vi "Initialize Offsets.vi"() -> (0 "Transactions":T1[](array[typedef]))   [LabVIEW 2013]
uses:
  Data Access Objects/Application/Number Of LBCBs.ctl
  Global Data/Transactions/Dataset Source.ctl
  Global Data/Transactions/Dataset Type.ctl
  Apps/Yes No Button.ctl
  Global Data/Transactions/Dataset Transaction Id.ctl
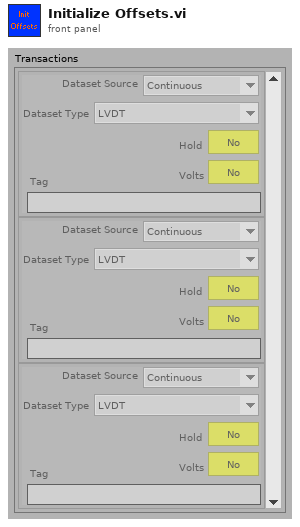
[diagram p1: front panel]
types:
  T1 = typedef "Dataset Transaction Id.ctl" = cluster{"Dataset Source":T2, "Dataset Type":T3, "Hold":T4, "Volts":T4, "Tag":string}
  T2 = typedef "Dataset Source.ctl" = enum16{"Continuous", "Hold", "ED", "Volts", "Offsets", "Increments"}
  T3 = typedef "Dataset Type.ctl" = enum16{"LVDT", "Load Cell", "Actuator Command", "Servo Error", "Displacement Command", "Displacement", "Force"}
  T4 = typedef "Yes No Button.ctl" = bool
  T5 = typedef "Number Of LBCBs.ctl" = enum16{"1", "2"}
  T6 = typedef "Dataset Source.ctl" = enum16{"Continuous", "Hold", "ED", "Volts", "Offsets"}
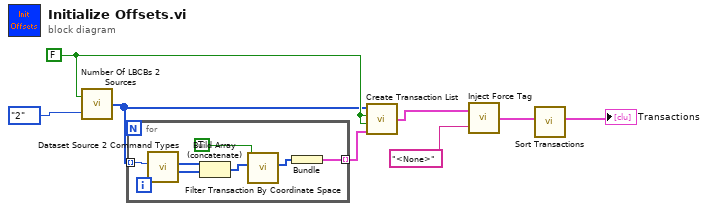
[diagram p0: block diagram]
diagram:
  w7 = FALSE ("Combined LBCBs")
  n1 = call "Number Of LBCBs 2 Sources.vi"("Number of LBCBs"=Number_Of_LBCBs."2", "Combined LBCBs"=w7) -> ("Sources"=w3:T6[])
  n2 = for {
    tunnel: w3 -> [w15] mode=indexing
    tunnel: [w9] -> w2 mode=indexing
    n3 = call "Dataset Source 2 Command Types.vi"("Dataset Source"=w15) -> ("No Command Types Out"=w13:T3[], "Command Types"=w14:T3[])  [unwired: 9 in]
    n4 = Build Array (concatenate)(w14, w13) -> (w12:T3[])
    n5 = call "Filter Transaction By Coordinate Space.vi"("Types In"=w12, "Coordinate Space"=TRUE) -> ("Types Out"=w10:T3[])  [unwired: 9 in]
    n6 = Bundle("Types Out"=w10) -> (w9:cluster{"Types Out":T3[]})  [unwired: 1 in]
  }
  n7 = call "Create Transaction List.vi"("Source Types"=w2, "Hold"=w7, "Volts"=w7, "Sources"=w3) -> ("Transactions"=w5:T1[])
  n8 = call "Inject Force Tag.vi"("Tag"="<None>", "Transactions In"=w5) -> ("Transactions Out"=w4:T1[])
  n9 = call "Sort Transactions.vi"("Transactions In"=w4) -> ("Transactions Out"=→"Transactions":T1[])  [unwired: 10 in]
